vi "UDP_LOOPBACK.vi"() -> ()   [LabVIEW 2012]
uses:
  Transport Layer/UDP Rx.lvclass
  Transport Layer/UDP Tx.lvclass
panel:
  in  "Stop Button":bool
  in  "Tx UDP Config":cluster{"Timeout":u16, "Local Port":u16}
  in  "Rx UDP Config":T1={"Local UDP Port (Tx)"=1002, "Remote IP (Rx)"="localhost", "Remote UDP Port (Rx)"=1234, "Timeout [ms]"=1}
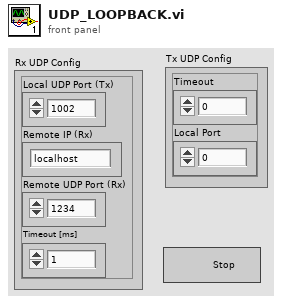
[diagram p1: front panel]
types:
  T1 = cluster{"Local UDP Port (Tx)":u16, "Remote IP (Rx)":string, "Remote UDP Port (Rx)":u16, "Timeout [ms]":u16}
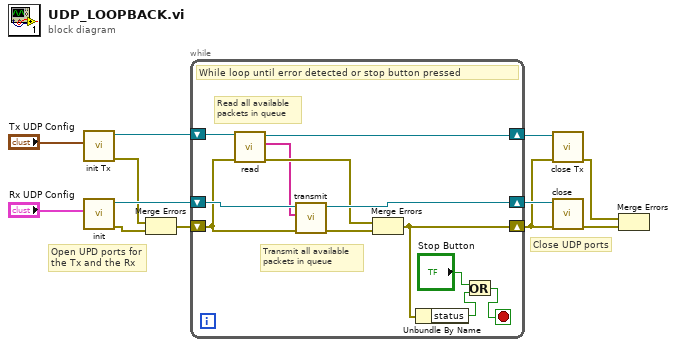
[diagram p0: block diagram]
diagram:
  # "Close UDP ports"
  # "Open UPD ports for\nthe Tx and the Rx"
  n1 = call "init Tx.vi"("Tx UDP config"="Tx UDP Config") -> ("error out"=w2:errorcluster, "UDP Tx.lvclass"=w10:refnum<class "UDP Tx.lvclass">)  [unwired: 9 in]
  n2 = call "init.vi"("Rx UDP Config"="Rx UDP Config") -> ("error out"=w1:errorcluster, "UDP Out"=w12:refnum<class "UDP Rx.lvclass">)  [unwired: 9 in]
  n3 = Merge Errors(w2, w1) -> (w3:errorcluster)
  n4 = while {
    shift-right: [w23] -> w11
    shift-left: w12 -> [w24]
    shift-right: [w21] -> w9
    shift-left: w10 -> [w22]
    shift-right: [w16] -> w6
    shift-left: w3 -> [w17]
    stop <- w15 stop-if-true
    # "Transmit all available\npackets in queue"
    # "Read all available\npackets in queue"
    # "While loop until error detected or stop button pressed"
    n5 = call "read.vi"("error in (no error)"=w17, "UDP Tx in"=w22) -> ("error out"=w20:errorcluster, "Received data"=w18:string[], "UDP Tx out"=w21:refnum<class "UDP Tx.lvclass">)  [unwired: 6 in, 1 out]
    n6 = call "transmit.vi"("error in (no error)"=w17, "Packets"=w18, "UDP in"=w24) -> ("error out"=w19:errorcluster, "UDP out"=w23:refnum<class "UDP Rx.lvclass">)  [unwired: 7 in]
    n7 = Merge Errors(w20, w19) -> (w16:errorcluster)
    n8 = Unbundle By Name(w16) -> ("status"=w14:bool)
    n9 = Or(x="Stop Button", y=w14) -> (x .or. y?=w15:bool)
  }
  n10 = call "close Tx.vi"("error in (no error)"=w6, "UDP Tx in"=w9) -> ("error out"=w8:errorcluster)  [unwired: 9 in]
  n11 = call "close.vi"("error in (no error)"=w6, "UDP in"=w11) -> ("error out"=w7:errorcluster)  [unwired: 9 in]
  n12 = Merge Errors(w8, w7) -> ()  [unwired: 1 out]
